vi "LoopselFF_1_or_2cam_eventdriven_CC3001.VI"() -> ()   [LabVIEW 2015]
uses:
  board.vis/Globals.vi
  <vilib>/Analysis/NI_AALBase.lvlib
panel:
  out "amount of devices":u8=1
  out "amount of cams":u8=1
  in  "CHB 8":bool
  in  "CHA 8":bool
  in  "CHB 7":bool
  in  "CHA 7":bool
  in  "CHB 6":bool
  in  "CHA 6":bool
  in  "CHB 5":bool
  in  "CHA 5":bool
  in  "CHB 4":bool
  in  "CHA 4":bool
  in  "CHB 3":bool
  in  "CHA 3":bool
  in  "CHB 2":bool
  in  "CHA 2":bool
  in  "CHB 1":bool
  in  "CHA 1":bool=TRUE
  in  "channel quick select (in hex)":u16=1 format="%x"
  out "tRMS":dbl=8.272957184592048 format="%0#.1f"
  out "mean":dbl=3064.5285285285286 format="%#_4f"
  in  "rms_pixel":u16=100
  in  "is FFT":bool=TRUE
  in  "IR gain":bool
  in  "continuous":bool=TRUE
  out "curr.block":u8=1
  out "Measure ON":bool
  in  "Board select\n1: board 1\n2: board 2\n3: both boards":u8=3
  in  "no.of blocks (nob)\npress enter":u32=1
  in  "block":u32(slide)=1 max=10 scale=0.9..1.0
  out "Signalverlaufgraph 2":u16[](graph)=[0, 0, 543, 543, 0, 1, 0, 0, 2, 2, 3, 3, 4, 4, 5, 5, 6, 6, 7, 7, 8, 8, 9, 9, 10, 10, 11, 11, 12, 12, 13, 13, 14, 14, 15, 15, 16, 16, 17, 17, 18, 18, 19, 19, 20, 20, 21, 21, 22, 22, 23, 23, 24, 24, 25, 25, 26, 26, 27, 27, 28, 28, 29, 29, 30, 30, 31, 31, 32, 32, 33, 33, 34, 34, 35, 35, 36, 36, 37, 37, 38, 38, 39, 39, 40, 40, 41, 41, 42, 42, 43, 43, 44, 44, 45, 45, 46, 46, 47, 47, 48, 48, 49, 49, 50, 50, 51, 51, 52, 52, 53, 53, 54, 54, 55, 55, 56, 56, 57, 57, 58, 58, 59, 59, 60, 60, 61, 61, 62, 62, 63, 63, 64, 64, 65, 65, 66, 66, 67, 67, 68, 68, 69, 69, 70, 70, 71, 71, 72, 72, 73, 73, 74, 74, 75, 75, 76, 76, 77, 77, 78, 78, 79, 79, 80, 80, 81, 81, 82, 82, 83, 83, 84, 84, 85, 85, 86, 86, 87, 87, 88, 88, 89, 89, 90, 90, 91, 91, 92, 92, 93, 93, 94, 94, 95, 95, 96, 96, 97, 97, 98, 98, 99, 99, 100, 100, 101, 101, 102, 102, 103, 103, 104, 104, 105, 105, 106, 106, 107, 107, 108, 108, 109, 109, 110, 110, 111, 111, 112, 112, 113, 113, 114, 114, 115, 115, 116, 116, 117, 117, 118, 118, 119, 119, 120, 120, 121, 121, 122, 122, 123, 123, 124, 124, 125, 125, 126, 126, 127, 127, 128, 128, 129, 129, 130, 130, 131, 131, 132, 132, 133, 133, 134, 134, 135, 135, 136, 136, 137, 137, 138, 138, 139, 139, 140, 140, 141, 141, 142, 142, 143, 143, 144, 144, 145, 145, 146, 146, 147, 147, 148, 148, 149, 149, 150, 150, 151, 151, 152, 152, 153, 153, 154, 154, 155, 155, 156, 156, 157, 157, 158, 158, 159, 159, 160, 160, 161, 161, 162, 162, 163, 163, 164, 164, 165, 165, 166, 166, 167, 167, 168, 168, 169, 169, 170, 170, 171, 171, 172, 172, 173, 173, 174, 174, 175, 175, 176, 176, 177, 177, 178, 178, 179, 179, 180, 180, 181, 181, 182, 182, 183, 183, 184, 184, 185, 185, 186, 186, 187, 187, 188, 188, 189, 189, 190, 190, 191, 191, 192, 192, 193, 193, 194, 194, 195, 195, 196, 196, 197, 197, 198, 198, 199, 199, 200, 200, 201, 201, 202, 202, 203, 203, 204, 204, 205, 205, 206, 206, 207, 207, 208, 208, 209, 209, 210, 210, 211, 211, 212, 212, 213, 213, 214, 214, 215, 215, 216, 216, 217, 217, 218, 218, 219, 219, 220, 220, 221, 221, 222, 222, 223, 223, 224, 224, 225, 225, 226, 226, 227, 227, 228, 228, 229, 229, 230, 230, 231, 231, 232, 232, 233, 233, 234, 234, 235, 235, 236, 236, 237, 237, 238, 238, 239, 239, 240, 240, 241, 241, 242, 242, 243, 243, 244, 244, 245, 245, 246, 246, 247, 247, 248, 248, 249, 249, 250, 250, 251, 251, 252, 252, 253, 253, 254, 254, 255, 255, 256, 256, 257, 257, 258, 258, 259, 259, 260, 260, 261, 261, 262, 262, 263, 263, 264, 264, 265, 265, 266, 266, 267, 267, 268, 268, 269, 269, 270, 270, 271, 271, 272, 272, 273, 273, 274, 274, 275, 275, 276, 276, 277, 277, 278, 278, 279, 279, 280, 280, 281, 281, 282, 282, 283, 283, 284, 284, 285, 285, 286, 286, 287, 287, 288, 288, 289, 289, 290, 290, 291, 291, 292, 292, 293, 293, 294, 294, 295, 295, 296, 296, 297, 297, 298, 298, 299, 299, 300, 300, 301, 301, 302, 302, 303, 303, 304, 304, 305, 305, 306, 306, 307, 307, 308, 308, 309, 309, 310, 310, 311, 311, 312, 312, 313, 313, 314, 314, 315, 315, 316, 316, 317, 317, 318, 318, 319, 319, 320, 320, 321, 321, 322, 322, 323, 323, 324, 324, 325, 325, 326, 326, 327, 327, 328, 328, 329, 329, 330, 330, 331, 331, 332, 332, 333, 333, 334, 334, 335, 335, 336, 336, 337, 337, 338, 338, 339, 339, 340, 340, 341, 341, 342, 342, 343, 343, 344, 344, 345, 345, 346, 346, 347, 347, 348, 348, 349, 349, 350, 350, 351, 351, 352, 352, 353, 353, 354, 354, 355, 355, 356, 356, 357, 357, 358, 358, 359, 359, 360, 360, 361, 361, 362, 362, 363, 363, 364, 364, 365, 365, 366, 366, 367, 367, 368, 368, 369, 369, 370, 370, 371, 371, 372, 372, 373, 373, 374, 374, 375, 375, 376, 376, 377, 377, 378, 378, 379, 379, 380, 380, 381, 381, 382, 382, 383, 383, 384, 384, 385, 385, 386, 386, 387, 387, 388, 388, 389, 389, 390, 390, 391, 391, 392, 392, 393, 393, 394, 394, 395, 395, 396, 396, 397, 397, 398, 398, 399, 399, 400, 400, 401, 401, 402, 402, 403, 403, 404, 404, 405, 405, 406, 406, 407, 407, 408, 408, 409, 409, 410, 410, 411, 411, 412, 412, 413, 413, 414, 414, 415, 415, 416, 416, 417, 417, 418, 418, 419, 419, 420, 420, 421, 421, 422, 422, 423, 423, 424, 424, 425, 425, 426, 426, 427, 427, 428, 428, 429, 429, 430, 430, 431, 431, 432, 432, 433, 433, 434, 434, 435, 435, 436, 436, 437, 437, 438, 438, 439, 439, 440, 440, 441, 441, 442, 442, 443, 443, 444, 444, 445, 445, 446, 446, 447, 447, 448, 448, 449, 449, 450, 450, 451, 451, 452, 452, 453, 453, 454, 454, 455, 455, 456, 456, 457, 457, 458, 458, 459, 459, 460, 460, 461, 461, 462, 462, 463, 463, 464, 464, 465, 465, 466, 466, 467, 467, 468, 468, 469, 469, 470, 470, 471, 471, 472, 472, 473, 473, 474, 474, 475, 475, 476, 476, 477, 477, 478, 478, 479, 479, 480, 480, 481, 481, 482, 482, 483, 483, 484, 484, 485, 485, 486, 486, 487, 487, 488, 488, 489, 489, 490, 490, 491, 491, 492, 492, 493, 493, 494, 494, 495, 495, 496, 496, 497, 497, 498, 498, 499, 499, 500, 500, 501, 501, 502, 502, 503, 503, 504, 504, 505, 505, 506, 506, 507, 507, 508, 508, 509, 509, 510, 510, 511, 511, 512, 512, 513, 513, 514, 514, 515, 515, 516, 516, 517, 517, 518, 518, 519, 519, 520, 520, 521, 521, 522, 522, 523, 523, 524, 524, 525, 525, 526, 526, 527, 527, 528, 528, 529, 529, 530, 530, 531, 531, 532, 532, 533, 533, 534, 534, 535, 535, 536, 536, 537, 537, 538, 538, 539, 539, 540, 540, 541, 541]
  out "Signalverlaufgraph":u16[](graph)=[2357, 2347, 2353, 2358, 0, 1, 0, 1, 2411, 2350, 2363, 2362, 2360, 34762, 35034, 35066, 35068, 35077, 35067, 35071, 35078, 35087, 35089, 35073, 35080, 35063, 35067, 35068, 35056, 35053, 35026, 35070, 35060, 35052, 35055, 35054, 35023, 35040, 35048, 35039, 35058, 35037, 35044, 35031, 35053, 35025, 35066, 35061, 35050, 35073, 35076, 35083, 35075, 35070, 35075, 35085, 35086, 35080, 35089, 35095, 35070, 35081, 35104, 35104, 35105, 35092, 35088, 35095, 35088, 35081, 35081, 35088, 35080, 35084, 35070, 35082, 35073, 35056, 35058, 35059, 35053, 35054, 35077, 35067, 35059, 35054, 35062, 35059, 35059, 35062, 35066, 35064, 35074, 35065, 35068, 35067, 35064, 35069, 35062, 35075, 35092, 35065, 35066, 35083, 35080, 35080, 35081, 35105, 35099, 35081, 35093, 35095, 35085, 35101, 35101, 35088, 35100, 35088, 35099, 35088, 35085, 35101, 35074, 35079, 35081, 35069, 35058, 35069, 35068, 35075, 35079, 35072, 35080, 35080, 35067, 35078, 35064, 35073, 35063, 35054, 35076, 35075, 35084, 35082, 35085, 35067, 35059, 35082, 35080, 35097, 35083, 35088, 35093, 35097, 35078, 35088, 35097, 35091, 35100, 35088, 35091, 35092, 35100, 35086, 35085, 35097, 35088, 35086, 35079, 35077, 35080, 35089, 35073, 35075, 35083, 35074, 35085, 35070, 35078, 35081, 35070, 35060, 35084, 35077, 35080, 35075, 35069, 35069, 35061, 35065, 35065, 35085, 35071, 35088, 35086, 35088, 35089, 35090, 35091, 35088, 35079, 35100, 35098, 35102, 35082, 35075, 35088, 35079, 35086, 35082, 35098, 35088, 35092, 35085, 35085, 35084, 35097, 35085, 35074, 35072, 35085, 35088, 35079, 35079, 35080, 35085, 35094, 35077, 35090, 35081, 35083, 35089, 35090, 35083, 35083, 35086, 35087, 35083, 35094, 35098, 35093, 35103, 35102, 35089, 35096, 35096, 35078, 35075, 35103, 35084, 35089, 35095, 35093, 35085, 35094, 35090, 35100, 35080, 35099, 35081, 35086, 35095, 35101, 35083, 35090, 35087, 35078, 35096, 35077, 35091, 35102, 35089, 35093, 35100, 35081, 35086, 35088, 35093, 35079, 35088, 35083, 35083, 35100, 35107, 35081, 35096, 35098, 35091, 35098, 35106, 35087, 35107, 35094, 35101, 35099, 35085, 35088, 35093, 35084, 35089, 35100, 35096, 35094, 35099, 35085, 35094, 35089, 35104, 35088, 35103, 35099, 35088, 35088, 35083, 35092, 35097, 35096, 35095, 35098, 35076, 35100, 35091, 35084, 35090, 35100, 35110, 35101, 35071, 35094, 35088, 35097, 35076, 35103, 35100, 35102, 35101, 35094, 35096, 35103, 35088, 35093, 35099, 35099, 35102, 35099, 35104, 35089, 35085, 35094, 35110, 35093, 35109, 35094, 35101, 35088, 35100, 35090, 35088, 35090, 35086, 35093, 35107, 35091, 35099, 35104, 35088, 35093, 35093, 35098, 35097, 35108, 35087, 35107, 35092, 35094, 35098, 35097, 35092, 35093, 35085, 35095, 35102, 35094, 35093, 35115, 35088, 35106, 35079, 35105, 35099, 35091, 35128, 35094, 35089, 35088, 35109, 35110, 35087, 35110, 35096, 35095, 35097, 35091, 35099, 35085, 35087, 35112, 35089, 35102, 35085, 35089, 35106, 35094, 35097, 35113, 35110, 35087, 35105, 35097, 35094, 35097, 35097, 35098, 35112, 35092, 35101, 35106, 35092, 35094, 35085, 35107, 35088, 35089, 35094, 35081, 35094, 35103, 35107, 35097, 35101, 35086, 35094, 35108, 35086, 35098, 35102, 35102, 35096, 35080, 35085, 35100, 35089, 35088, 35104, 35112, 35100, 35102, 35102, 35097, 35106, 35099, 35081, 35097, 35101, 35109, 35100, 35114, 35098, 35092, 32940, 29697, 29585, 29528, 29434, 29346, 29303, 29248, 29143, 29102, 29112, 29035, 28966, 28956, 28848, 28789, 28725, 28651, 28612, 28562, 28516, 28427, 28371, 28320, 28264, 28200, 28178, 28101, 28056, 27957, 27925, 27901, 27776, 27758, 27701, 27631, 27579, 27545, 27475, 27425, 27382, 27318, 27302, 27222, 27176, 27114, 27069, 27020, 26974, 26944, 26887, 26793, 26807, 26744, 26714, 26624, 26586, 26540, 26466, 26393, 26379, 26282, 26220, 26157, 26029, 25929, 25768, 25543, 2252, 2400, 2386, 2390, 2368, 2373, 2377, 2379, 2379, 2378, 2377, 2380, 2373, 2379, 2386, 2383, 2376, 2381, 2378, 2377, 2376, 2373, 2385, 2377, 2381, 2376, 2379, 2379, 2376, 2376, 2376, 2379, 2384, 2378, 2374, 2380, 2377, 2381, 2380, 2371, 2379, 2376, 2379, 2384, 2380, 2380, 2377, 2368, 2376, 2375, 2378, 2370, 2374, 2375, 2383, 2372, 2379, 2374, 2381, 2369, 2375, 2368, 2373, 2368, 2368, 2372, 2374, 2371, 2368, 2373, 2372, 2370, 2372, 2374, 2375, 2367, 2367, 2370, 2369, 2375, 2372, 2373, 2378, 2372, 2366, 2372, 2370, 2374, 2365, 2373, 2375, 2374, 2370, 2370, 2369, 2369, 2374, 2371, 2373, 2371, 2372, 2371, 2366, 2368, 2370, 2362, 2370, 2372, 2366, 2374, 2369, 2368, 2371, 2368, 2365, 2362, 2375, 2373, 2369, 2366, 2367, 2371, 2362, 2377, 2371, 2367, 2369, 2366, 2371, 2366, 2364, 2366, 2360, 2365, 2374, 2362, 2371, 2373, 2366, 2364, 2367, 2364, 2368, 2360, 2360, 2363, 2367, 2368, 2367, 2371, 2364, 2368, 2366, 2359, 2363, 2365, 2368, 2368, 2358, 2357, 2365, 2364, 2369, 2362, 2364, 2364, 2363, 2358, 2363, 2364, 2359, 2360, 2358, 2370, 2358, 2361, 2363, 2355, 2361, 2369, 2363, 2366, 2365, 2368, 2363, 2360, 2359, 2361, 2359, 2363, 2356, 2365, 2362, 2360, 2368, 2362, 2366, 2370, 2358, 2366, 2364, 2366, 2362, 2363, 2356, 2365, 2363, 2361, 2363, 2367, 2366, 2365, 2357, 2366, 2359, 2361, 2360, 2360, 2363, 2365, 2364, 2360, 2360, 2357, 2355, 2362, 2361, 2361, 2364, 2364, 2361, 2364, 2361, 2363, 2358, 2363, 2357, 2355, 2357, 2365, 2357, 2367, 2365, 2363, 2354, 2360, 2356, 2358, 2362, 2359, 2360, 2362, 2362, 2355, 2360, 2360, 2360, 2361, 2360, 2359, 2357, 2364, 2359, 2361, 2362, 2360, 2359, 2360, 2355, 2355, 2362, 2358, 2358, 2357, 2357, 2360, 2360, 2363, 2353, 2353, 2358, 2358, 2358, 2362, 2360, 2362, 2359, 2356, 2357, 2360, 2355, 2353, 2360, 2362, 2358, 2358, 2350, 2357, 2362, 2354, 2354, 2356, 2360, 2360, 2355, 2361, 2354, 2360, 2356, 2355, 2355, 2362, 2359, 2362, 2363, 2359, 2361, 2358, 2355, 2356, 2354, 2358, 2364, 2356, 2362, 2358, 2354, 2360, 2362, 2361, 2358, 2361, 2362, 2358, 2363, 2359, 2363, 2364, 2356, 2357, 2356, 2354, 2360, 2357, 2355, 2359, 2358, 2356, 2362, 2360, 2357, 2359, 2357, 2357, 2355, 2357, 2357, 2357, 2364, 2360, 2355, 2358, 2355, 2357, 2360, 2353, 2355, 2352, 2362, 2354, 2355, 2360, 2357, 2352, 2359, 2356, 2356, 2358, 2353, 2357, 2356, 2355, 2349, 2361, 2358, 2354, 2358, 2359, 2355, 2360, 2354, 2357, 2357, 2353, 2354, 2359, 2359, 2355, 2349, 2358, 2358, 2355, 2353, 2353, 2357, 2357, 2357, 2354, 2358, 2359, 2354, 2353, 2352, 2358, 2361, 2357, 2350, 2350, 2352, 2360, 2351, 2355, 2354, 2360, 2357, 2355, 2355, 2355, 2350, 2357, 2357, 2358, 2358, 2356, 2353, 2352, 2354, 2353, 2357, 2357, 2353, 2358, 2360, 2361, 2355, 2357, 2361, 2357, 2358, 2356, 2355, 2358, 2354, 2351, 2355, 2352, 2354, 2352, 2354, 2363, 2359, 2358, 2357, 2349, 2358, 2352, 2356, 2355, 2359, 2353, 2353, 2361, 2359, 2359, 2357, 2357, 2349, 2353, 2353, 2350, 2358, 2357, 2356, 2358, 2356, 2356, 2355, 2355, 2355, 2351, 2355, 2357, 2352, 2354, 2348, 2354, 2348, 2354, 2350, 2352, 2353, 2359, 2356, 2351, 2356, 2357, 2352, 2354, 2355, 2359, 2353, 2354, 2352, 2349, 2362, 2353, 2360, 2349, 2357, 2352, 2359, 2348, 2359, 2349, 2358, 2348, 2349, 2351, 2356, 2353, 2358, 2353, 2354, 2360, 2355, 2356, 2358, 2348, 2351, 2354, 2358, 2360, 2360, 2359, 2356, 2356, 2354, 2357, 2350, 2351, 2351]
  out "boards recognised":u8=1
  in  "alloc mem":bool
  out "FREE \nRAM MB":dbl=14941.0
  out "BUILT-IN\nRAM MB":dbl=18096.0
  out "SEC":dbl=5.9999999999999995e-05
  out "MB RAM":dbl
  in  "pos slope":u8=1
  in  "both slopes":u8
  in  "DAT in 10ns":u32
  in  "extTrig  0/1\n0 : internal\n1:  \"I\" input (laser)":u8
  in  "stop all":bool
  in  "start":bool
  in  "sample":u32(slide)=2 max=3000 scale=0.9..110.0
  in  "no.of samples (nos)":u32=3000
  in  "exposuretime[ms]":dbl=1.0 format="%.3f"
  # "Camera Control 1"
  # "Camera Control 5"
  # "Start with run"
  # "Abort with ESC"
  # "Camera Control 6"
  # "Camera Control 2"
  # "Camera Control 3"
  # "Camera Control 7"
  # "Camera Control 4"
  # "Camera Control 8"
  # "press Esc to stop measurement"
  # "exit here"
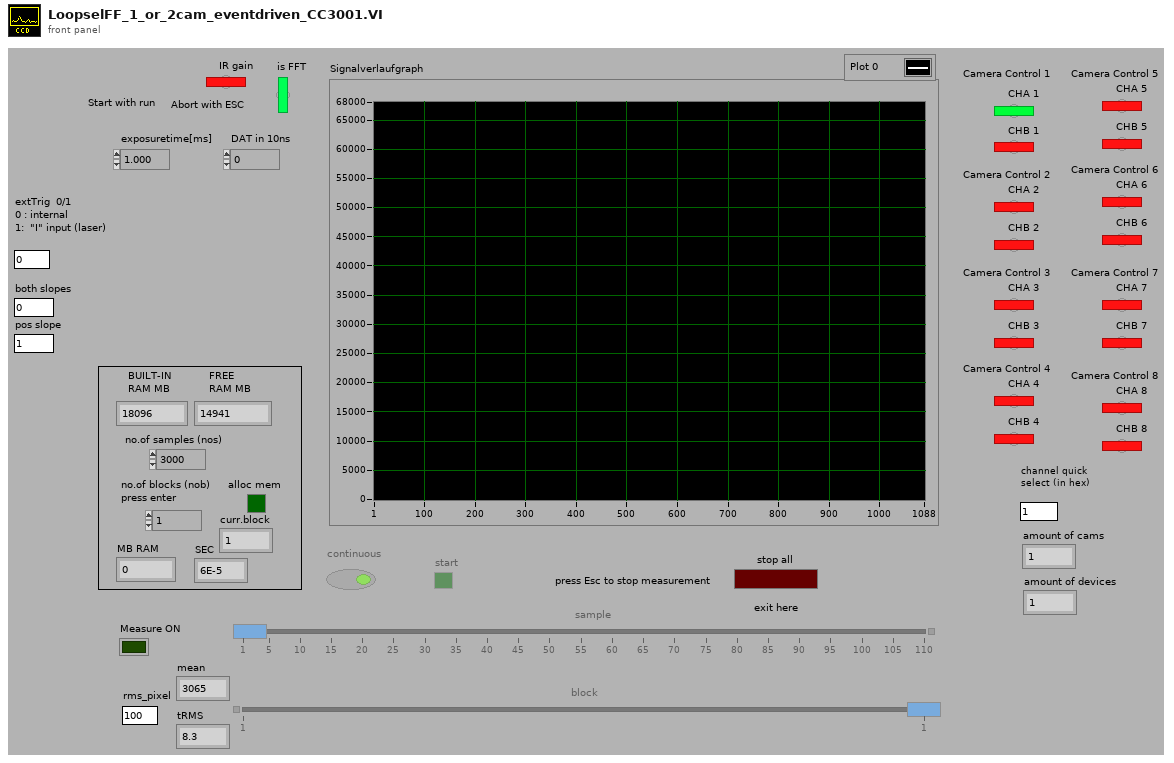
[diagram p1: front panel]
types:
  T1 = enum8{"Enabled", "Disabled", "Disabled and Grayed Out"}
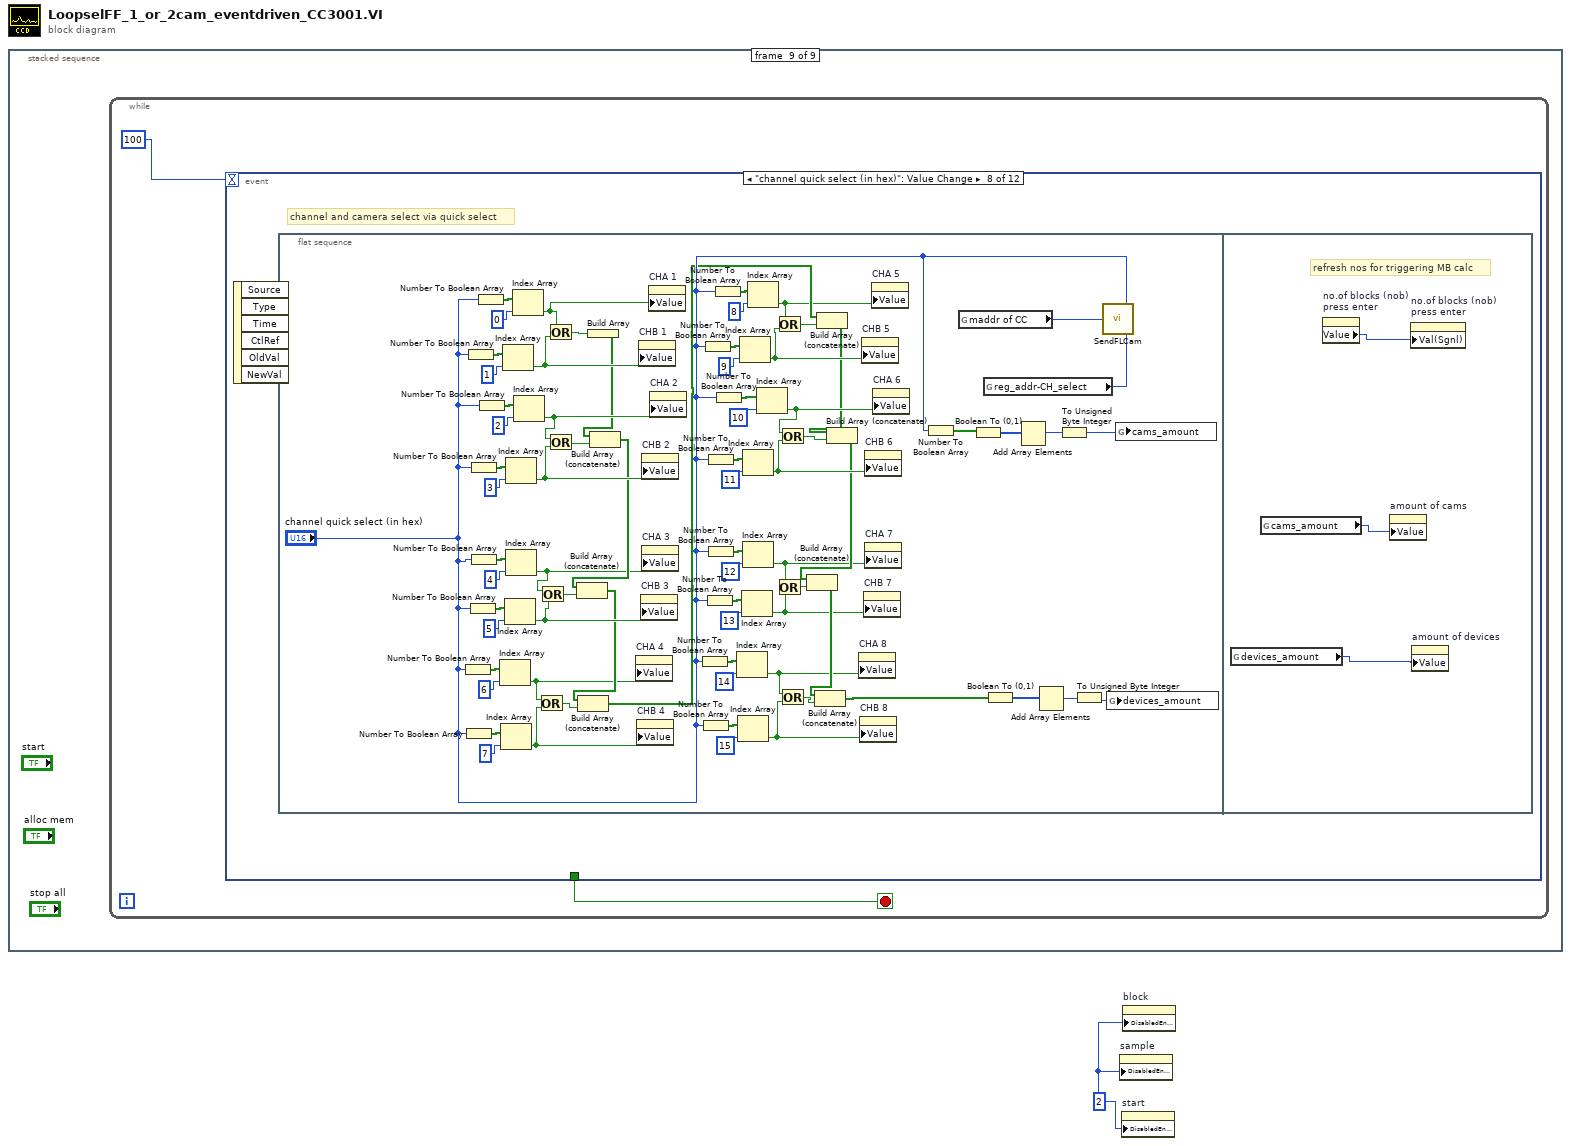
[diagram p0: block diagram]
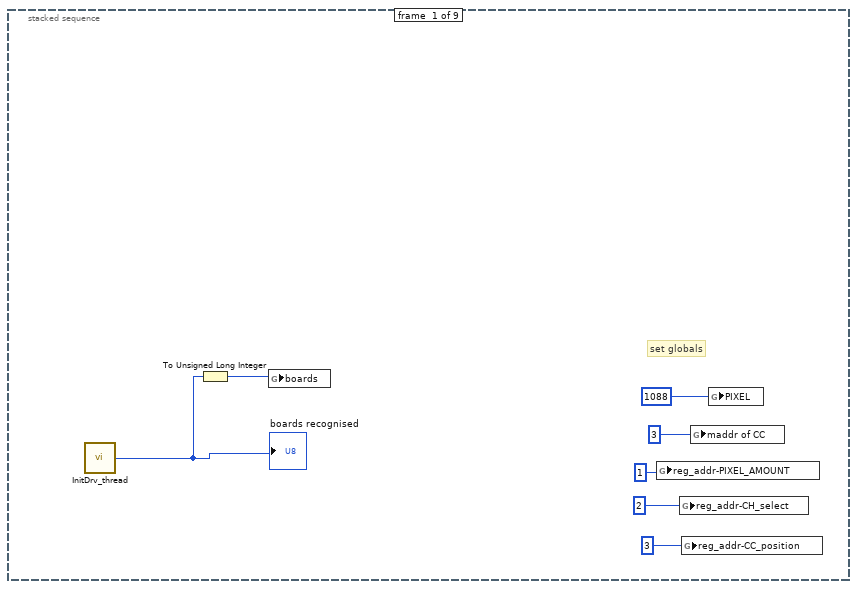
[diagram p2: hidden frame]
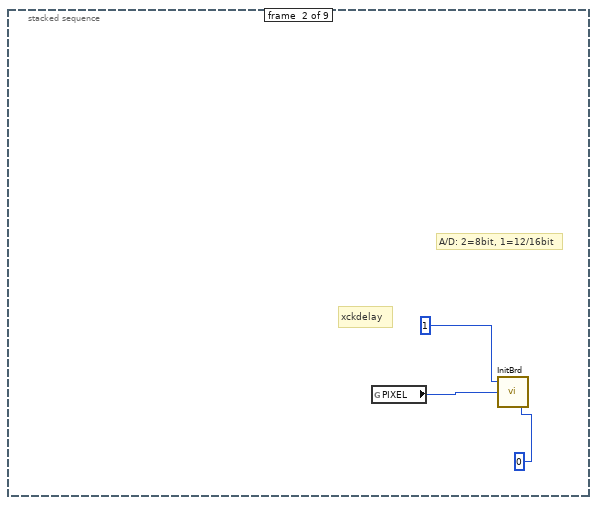
[diagram p3: hidden frame]
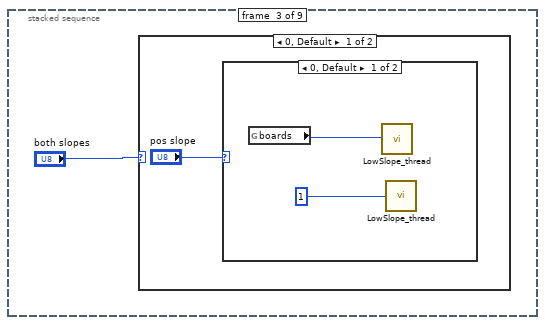
[diagram p4: hidden frame]
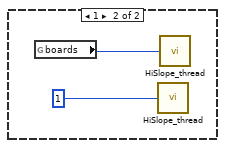
[diagram p5: hidden frame]
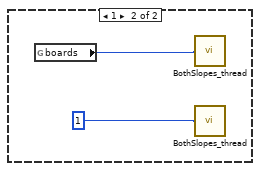
[diagram p6: hidden frame]
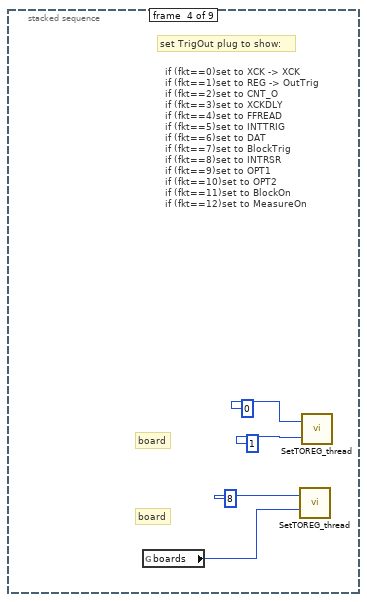
[diagram p7: hidden frame]
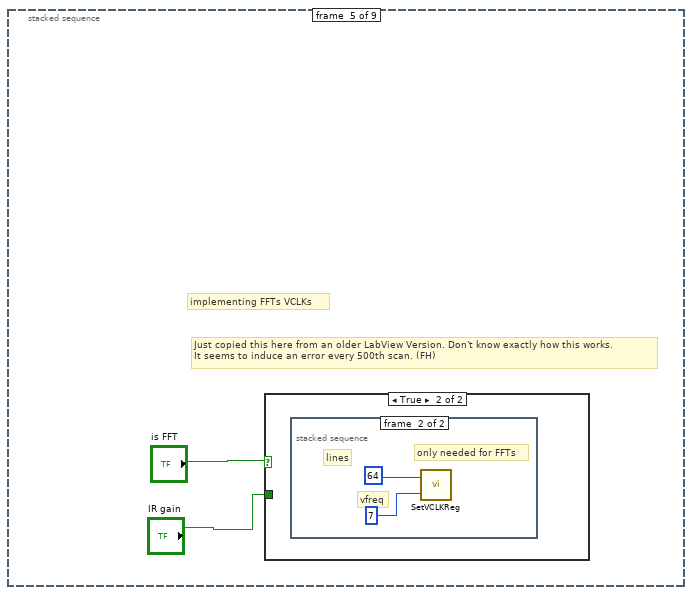
[diagram p8: hidden frame]
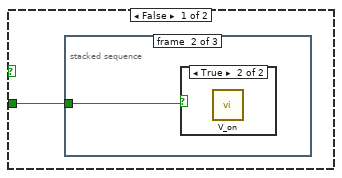
[diagram p9: hidden frame]
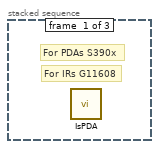
[diagram p10: hidden frame]
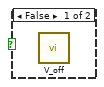
[diagram p11: hidden frame]
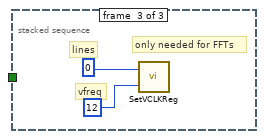
[diagram p12: hidden frame]
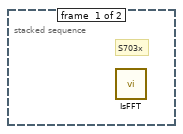
[diagram p13: hidden frame]
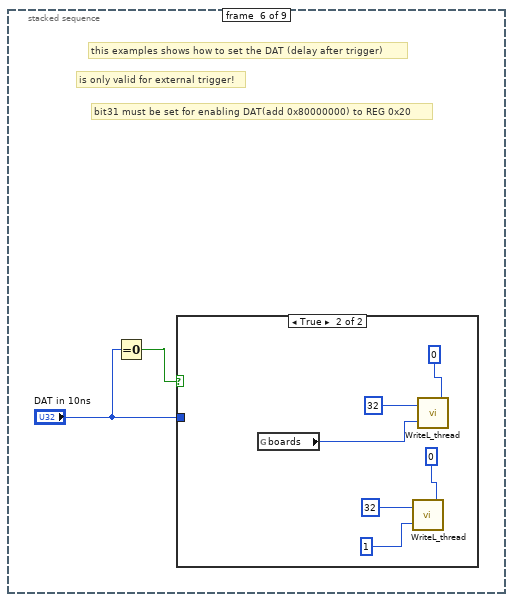
[diagram p14: hidden frame]
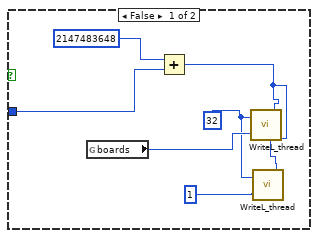
[diagram p15: hidden frame]
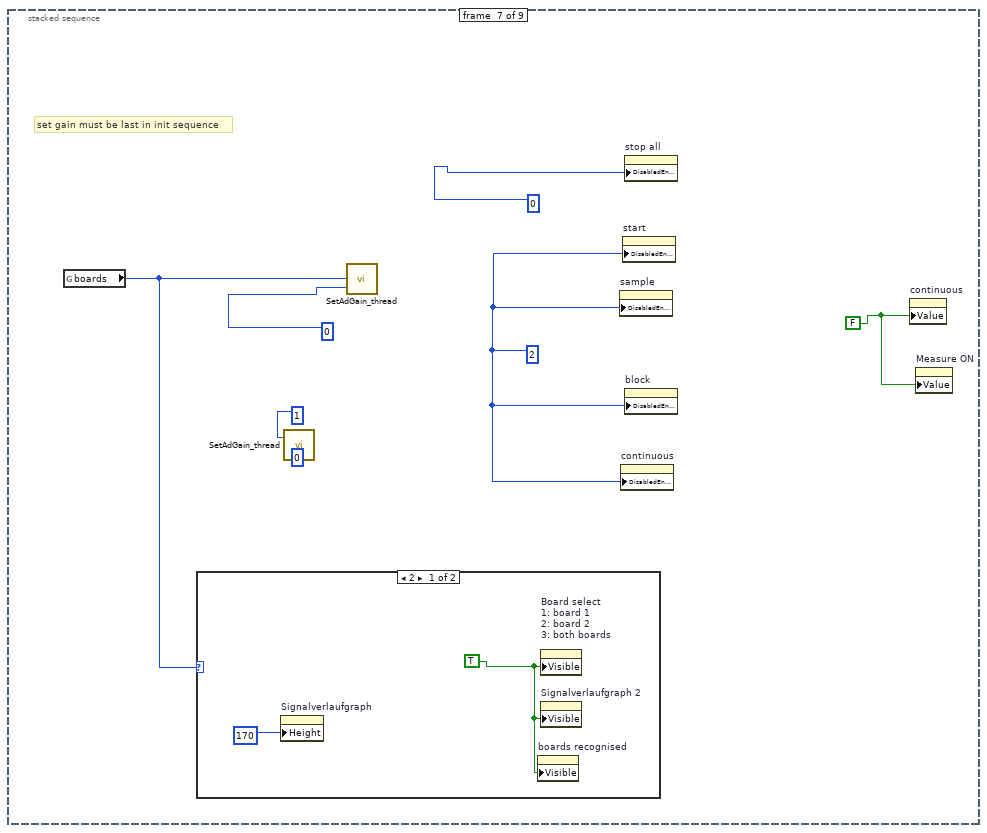
[diagram p16: hidden frame]
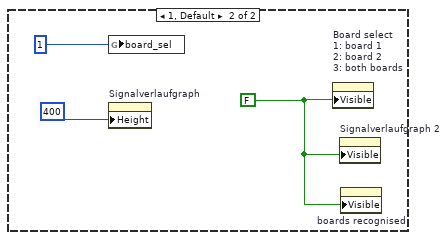
[diagram p17: hidden frame]
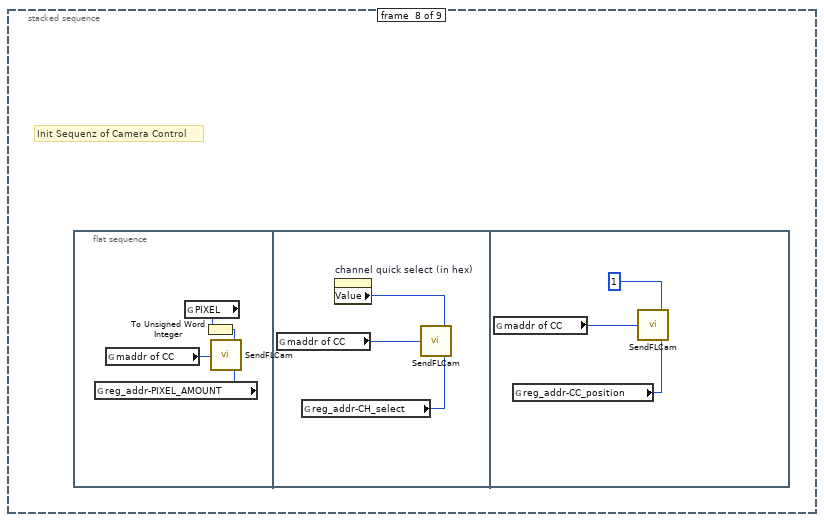
[diagram p18: hidden frame]
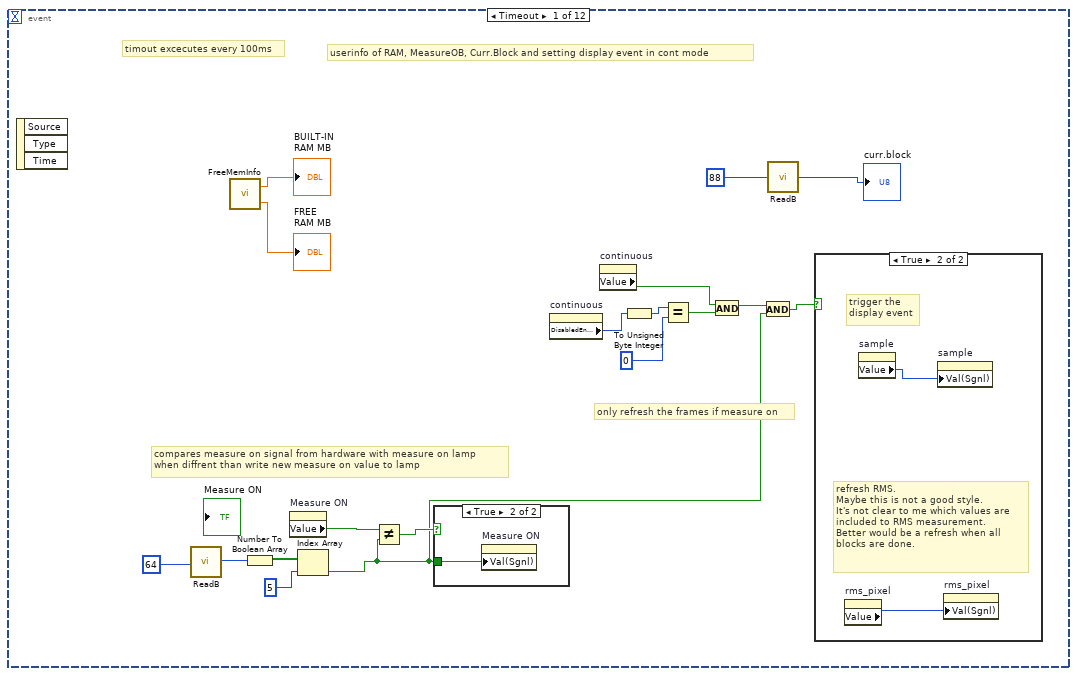
[diagram p19: hidden frame]
diagram:
  w1 = 2
  n1 = stacked-sequence {
    frame #0 {
      # "set globals"
      n2 = call "InitDrv_thread.vi"() -> ("Boards"=w6:u8)  [unwired: 1 in]
      "boards recognised" <- w6
      n3 = To Unsigned Long Integer(number=w6) -> (unsigned 32bit integer=w7:u32)
      n4 = global write "Globals.vi" "boards"(w7) -> ()
      n5 = global write "Globals.vi" "reg_addr-PIXEL_AMOUNT"(u8 1) -> ()
      n6 = global write "Globals.vi" "reg_addr-CH_select"(u8 2) -> ()
      n7 = global write "Globals.vi" "reg_addr-CC_position"(u8 3) -> ()
      n8 = global write "Globals.vi" "maddr of CC"(u8 3) -> ()
      n9 = global write "Globals.vi" "PIXEL"(u32 1088) -> ()
    }
    frame #1 {
      # "xckdelay"
      # "A/D: 2=8bit, 1=12/16bit"
      n10 = global read "Globals.vi" "PIXEL"() -> (w11:u32)
      n11 = call "InitBrd.vi"("xckdly"=u32 0, "pixel"=w11, "flag816"=u32 1) -> ()  [unwired: 3 in]
    }
    frame #2 {
      n12 = case shown="0, Default" "both slopes" {
        frame 0, Default {
          n13 = case shown="0, Default" "pos slope" {
            frame 0, Default {
              n14 = global read "Globals.vi" "boards"() -> (w14:u32)
              n15 = call "LowSlope_thread.vi"("board"=w14) -> ()  [unwired: 1 in]
              n16 = call "LowSlope_thread.vi"("board"=1) -> ()  [unwired: 1 in]
            }
            frame 1 {
              n17 = global read "Globals.vi" "boards"() -> (w17:u32)
              n18 = call "HiSlope_thread.vi"("board"=1) -> ()  [unwired: 1 in]
              n19 = call "HiSlope_thread.vi"("board"=w17) -> ()  [unwired: 1 in]
            }
          }
        }
        frame 1 {
          n20 = global read "Globals.vi" "boards"() -> (w19:u32)
          n21 = call "BothSlopes_thread.vi"("board"=w19) -> ()  [unwired: 1 in]
          n22 = call "BothSlopes_thread.vi"("board"=1) -> ()  [unwired: 1 in]
        }
      }
    }
    frame #3 {
      # "board"
      # "board"
      # "set TrigOut plug to show:"
      # "if (fkt==0)set to XCK -> XCK\nif (fkt==1)set to REG -> OutTrig\nif (fkt==2)set to CNT_O\nif (fkt==3)set to XCKDLY\nif (fkt==4)set to FFREAD\nif (fkt==5)set to INTTRIG\nif (fkt==6)set to DAT\nif (fkt==7)set to BlockTrig\nif (fkt==8)set to INTRSR\nif (fkt==9)set to OPT1\nif (fkt==10)set to OPT2\nif (fkt==11)set to BlockOn\nif (fkt==12)set to MeasureOn"
      n23 = global read "Globals.vi" "boards"() -> (w23:u32)
      n24 = call "SetTOREG_thread.vi"("board"=w23, "fkt"=u8 8) -> ()  [unwired: 1 in]
      n25 = call "SetTOREG_thread.vi"("board"=u32 1, "fkt"=u8 0) -> ()  [unwired: 1 in]
    }
    frame #4 {
      # "implementing FFTs VCLKs"
      # "Just copied this here from an older LabView Version. Don't know exactly how this works.\nIt seems to induce an error every 500th scan. (FH)"
      n26 = case shown="True" "is FFT" {
        tunnel: "IR gain" -> [w26 _]
        frame False {
          n27 = stacked-sequence {
            tunnel: w26 -> [_ w27 _]
            frame #0 {
              # "For IRs G11608"
              # "For PDAs S390x"
              n28 = call "IsPDA.vi"() -> ()  [unwired: 1 in]
            }
            frame #1 {
              n29 = case shown="True" w27 {
                frame False {
                  n30 = call "V_off.vi"() -> ()  [unwired: 1 in]
                }
                frame True {
                  n31 = call "V_on.vi"() -> ()  [unwired: 1 in]
                }
              }
            }
            frame #2 {
              # "only needed for FFTs"
              # "vfreq"
              # "lines"
              n32 = call "SetVCLKReg.vi"("vfreq"=u8 12, "lines"=u32 0) -> ()  [unwired: 1 in]
            }
          }
        }
        frame True {
          n33 = stacked-sequence {
            frame #0 {
              # "S703x"
              n34 = call "IsFFT.vi"() -> ()  [unwired: 1 in]
            }
            frame #1 {
              # "only needed for FFTs"
              # "vfreq"
              # "lines"
              n35 = call "SetVCLKReg.vi"("vfreq"=u8 7, "lines"=u32 64) -> ()  [unwired: 1 in]
            }
          }
        }
      }
    }
    frame #5 {
      # "bit31 must be set for enabling DAT(add 0x80000000) to REG 0x20"
      # "is only valid for external trigger!"
      # "this examples shows how to set the DAT (delay after trigger)"
      n36 = Equal To 0?(x="DAT in 10ns") -> (x = 0?=w33:bool)
      n37 = case shown="True" w33 {
        tunnel: "DAT in 10ns" -> [w38 _]
        frame False {
          w35 = u32 32
          n38 = global read "Globals.vi" "boards"() -> (w37:u32)
          n39 = Add(x=u32 2147483648, y=w38) -> (x+y=w36:u32)
          n40 = call "WriteL_thread.vi"("val"=w36, "board"=w37, "offset"=w35) -> ()
          n41 = call "WriteL_thread.vi"("val"=w36, "board"=u32 1, "offset"=w35) -> ()
        }
        frame True {
          n42 = global read "Globals.vi" "boards"() -> (w44:u32)
          n43 = call "WriteL_thread.vi"("val"=u32 0, "board"=u32 1, "offset"=u32 32) -> ()
          n44 = call "WriteL_thread.vi"("val"=u32 0, "board"=w44, "offset"=u32 32) -> ()
        }
      }
    }
    frame #6 {
      w46 = FALSE
      w52 = 2
      # "set gain must be last in init sequence"
      n45 = global read "Globals.vi" "boards"() -> (w50:u32)
      n46 = case shown="2" w50 {
        frame 2 {
          w54 = TRUE
          n47 = property on="Signalverlaufgraph" class="WFGraph (strict)"("Height"=u8 170) -> ()  [unwired: 2 in, 2 out]
          n48 = property on="boards recognised" class="DigNum (strict)"("Visible"=w54) -> ()  [unwired: 2 in, 2 out]
          n49 = property on="Board select\n1: board 1\n2: board 2\n3: both boards" class="DigNum (strict)"("Visible"=w54) -> ()  [unwired: 2 in, 2 out]
          n50 = property on="Signalverlaufgraph 2" class="WFGraph (strict)"("Visible"=w54) -> ()  [unwired: 2 in, 2 out]
        }
        frame 1, Default {
          w55 = FALSE
          n51 = global write "Globals.vi" "board_sel"(u8 1) -> ()
          n52 = property on="Signalverlaufgraph" class="WFGraph (strict)"("Height"=400) -> ()  [unwired: 2 in, 2 out]
          n53 = property on="Board select\n1: board 1\n2: board 2\n3: both boards" class="DigNum (strict)"("Visible"=w55) -> ()  [unwired: 2 in, 2 out]
          n54 = property on="Signalverlaufgraph 2" class="WFGraph (strict)"("Visible"=w55) -> ()  [unwired: 2 in, 2 out]
          n55 = property on="boards recognised" class="DigNum (strict)"("Visible"=w55) -> ()  [unwired: 2 in, 2 out]
        }
      }
      n56 = call "SetAdGain_thread.vi"("gain"=u8 0, "board"=u32 1) -> ()  [unwired: 1 in]
      n57 = call "SetAdGain_thread.vi"("gain"=u8 0, "board"=w50) -> ()  [unwired: 1 in]
      n58 = property on="sample" class="Slide (strict)"("DisabledEnum"=w52) -> ()  [unwired: 2 in, 2 out]
      n59 = property on="continuous" class="Bool (strict)"("DisabledEnum"=w52) -> ()  [unwired: 2 in, 2 out]
      n60 = property on="start" class="Bool (strict)"("DisabledEnum"=w52) -> ()  [unwired: 2 in, 2 out]
      n61 = property on="stop all" class="Bool (strict)"("DisabledEnum"=0) -> ()  [unwired: 2 in, 2 out]
      n62 = property on="block" class="Slide (strict)"("DisabledEnum"=w52) -> ()  [unwired: 2 in, 2 out]
      n63 = property on="continuous" class="Bool (strict)"("Value"=w46) -> ()  [unwired: 2 in, 2 out]
      n64 = property on="Measure ON" class="Bool (strict)"("Value"=w46) -> ()  [unwired: 2 in, 2 out]
    }
    frame #7 {
      # "Init Sequenz of Camera Control"
      n65 = flat-sequence {
        frame #0 {
          n66 = global read "Globals.vi" "reg_addr-PIXEL_AMOUNT"() -> (w61:u8)
          n67 = global read "Globals.vi" "maddr of CC"() -> (w60:u8)
          n68 = global read "Globals.vi" "PIXEL"() -> (w59:u32)
          n69 = To Unsigned Word Integer(number=w59) -> (unsigned 16bit integer=w58:u16)
          n70 = call "SendFLCam.vi"("madr"=w60, "data"=w58, "adadr"=w61) -> ()
        }
        frame #1 {
          n71 = global read "Globals.vi" "maddr of CC"() -> (w64:u8)
          n72 = global read "Globals.vi" "reg_addr-CH_select"() -> (w63:u8)
          n73 = property on="channel quick select (in hex)" class="DigNum (strict)"() -> ("Value"=w62:u16)  [unwired: 2 in, 2 out]
          n74 = call "SendFLCam.vi"("madr"=w64, "data"=w62, "adadr"=w63) -> ()
        }
        frame #2 {
          n75 = global read "Globals.vi" "maddr of CC"() -> (w67:u8)
          n76 = global read "Globals.vi" "reg_addr-CC_position"() -> (w66:u8)
          n77 = call "SendFLCam.vi"("madr"=w67, "data"=u16 1, "adadr"=w66) -> ()
        }
      }
    }
    frame #8 {
      n78 = while {
        stop <- w69 stop-if-true
        n79 = event shown="[7] \"channel quick select (in hex)\": Value Change" {
          selector: _ -> [_ _ _ _ _ _ _ _ _ _ _ _]
          dyn-events: _ -> [_ _ _ _ _ _ _ _ _ _ _ _]
          timeout: 100 -> [_ _ _ _ _ _ _ _ _ _ _ _]
          tunnel: [_ _ _ _ _ _ _ _ _ _ w318 _] -> w69
          event Timeout {
            # "only refresh the frames if measure on"
            # "compares measure on signal from hardware with measure on lamp\nwhen diffrent than write new measure on value to lamp"
            # "timout excecutes every 100ms"
            # "userinfo of RAM, MeasureOB, Curr.Block and setting display event in cont mode"
            n80 = event-data() -> ()  [unwired: 1 in, 3 out]
            n81 = call "ReadB.vi"("Offset"=u32 64) -> ("Data"=w84:u8)
            n82 = call "FreeMemInfo.vi"() -> ("PhysicalSpace"=→"BUILT-IN\nRAM MB":dbl, "PhysicalFreeSpace"=→"FREE \nRAM MB":dbl)  [unwired: 1 in]
            n83 = Number To Boolean Array(number=w84) -> (Boolean array=w83:bool[])
            n84 = property on="Measure ON" class="Bool (strict)"() -> ("Value"=w77:bool)  [unwired: 2 in, 2 out]
            n85 = Index Array(array=w83, index=5) -> (element=w73:bool)
            n86 = Not Equal?(x=w77, y=w73) -> (x != y?=w76:bool)
            n87 = case shown="True" w76 {
              tunnel: w73 -> [_ w88]
              frame False {
              }
              frame True {
                n88 = property on="Measure ON" class="Bool (strict)"("Val(Sgnl)"=w88) -> ()  [unwired: 2 in, 2 out]
              }
            }
            n89 = property on="continuous" class="Bool (strict)"() -> ("DisabledEnum"=w70:T1)  [unwired: 2 in, 2 out]
            n90 = property on="continuous" class="Bool (strict)"() -> ("Value"=w79:bool)  [unwired: 2 in, 2 out]
            n91 = To Unsigned Byte Integer(number=w70) -> (unsigned 8bit integer=w71:u8)
            n92 = Equal?(x=w71, y=u8 0) -> (x = y?=w78:bool)
            n93 = And(x=w79, y=w78) -> (x .and. y?=w75:bool)
            n94 = And(x=w75, y=w73) -> (x .and. y?=w74:bool)
            n95 = call "ReadB.vi"("Offset"=u32 88) -> ("Data"=→"curr.block":u8)
            n96 = case shown="True" w74 {
              frame False {
              }
              frame True {
                # "refresh RMS.\nMaybe this is not a good style.\nIt's not clear to me which values are \nincluded to RMS measurement.\nBetter would be a refresh when all\nblocks are done."
                # "trigger the \ndisplay event"
                n97 = property on="rms_pixel" class="DigNum (strict)"() -> ("Value"=w89:u16)  [unwired: 2 in, 2 out]
                n98 = property on="sample" class="Slide (strict)"() -> ("Value"=w90:u32)  [unwired: 2 in, 2 out]
                n99 = property on="sample" class="Slide (strict)"("Val(Sgnl)"=w90) -> ()  [unwired: 2 in, 2 out]
                n100 = property on="rms_pixel" class="DigNum (strict)"("Val(Sgnl)"=w89) -> ()  [unwired: 2 in, 2 out]
              }
            }
          }
          event "Measure ON": Value Change {
            # "triggers on value change of measure on. this happens on start of measurement and after measurement\nwhen continuous: not after finishing all blocks, only when exiting measurement"
            n101 = event-data() -> ("NewVal"=w91:bool)  [unwired: 1 in, 5 out]
            n102 = property on="continuous" class="Bool (strict)"() -> ("Value"=w92:bool)  [unwired: 2 in, 2 out]
            n103 = And(x=w92, y=w91) -> (x .and. y?=w93:bool)
            n104 = case shown="False" w91 {
              frame False {
                n105 = property on="stop all" class="Bool (strict)"("DisabledEnum"=0) -> ()  [unwired: 2 in, 2 out]
              }
              frame True {
              }
            }
            n106 = case shown="True" w93 {
              frame False {
              }
              frame True {
                n107 = property on="stop all" class="Bool (strict)"("DisabledEnum"=2) -> ()  [unwired: 2 in, 2 out]
              }
            }
          }
          event "Board select\n1: board 1\n2: board 2\n3: both boards": Value Change {
            # "selecting number of cams"
            n108 = event-data() -> ()  [unwired: 1 in, 6 out]
            n109 = global read "Globals.vi" "boards"() -> (w96:u32)
            n110 = case shown="2" w96 {
              frame 0, Default {
              }
              frame 2 {
                n111 = global write "Globals.vi" "board_sel"("Board select\n1: board 1\n2: board 2\n3: both boards") -> ()
              }
            }
          }
          event "continuous": Value Change {
            # "setting continuos mode"
            n112 = event-data() -> ()  [unwired: 1 in, 6 out]
            n113 = case shown="False" "continuous" {
              tunnel: [u8 0 u8 1] -> w98
              frame False {
              }
              frame True {
              }
            }
            n114 = call "contFFLoop.vi"("Numeric"=w98) -> ()  [unwired: 1 in]
          }
          event "alloc mem": Value Change {
            w108 = 0
            # "update params"
            # "Setup DMA"
            n115 = event-data() -> ()  [unwired: 1 in, 6 out]
            n116 = global read "Globals.vi" "cams_amount"() -> (w105:u8)
            n117 = global read "Globals.vi" "nob"() -> (w106:u32)
            n118 = global read "Globals.vi" "nos"() -> (w107:u32)
            n119 = To Unsigned Long Integer(number=w105) -> (unsigned 32bit integer=w104:u32)
            n120 = global read "Globals.vi" "boards"() -> (w111:u32)
            n121 = Multiply(x=w104, y=w106) -> (x*y=w102:u32)
            n122 = Multiply(x=w104, y=w107) -> (x*y=w103:u32)
            n123 = case shown="2" w111 {
              selector: w111 -> [_ w112]
              tunnel: w103 -> [_ w113]
              tunnel: w102 -> [_ w114]
              frame 1, Default {
              }
              frame 2 {
                # "Setup DMA"
                n124 = call "SetupDMA_thread.vi"("blocks"=w114, "nos"=w113, "Drv"=w112) -> ()  [unwired: 2 in]
              }
            }
            n125 = call "SetupDMA_thread.vi"("blocks"=w102, "nos"=w103, "Drv"=u32 1) -> ()  [unwired: 2 in]
            n126 = property on="continuous" class="Bool (strict)"("DisabledEnum"=w108) -> ()  [unwired: 2 in, 2 out]
            n127 = property on="block" class="Slide (strict)"("DisabledEnum"=w108) -> ()  [unwired: 2 in, 2 out]
            n128 = property on="sample" class="Slide (strict)"("DisabledEnum"=w108) -> ()  [unwired: 2 in, 2 out]
            n129 = property on="exposuretime[ms]" class="DigNum (strict)"() -> ("Value"=w110:dbl)  [unwired: 2 in, 2 out]
            n130 = property on="start" class="Bool (strict)"("DisabledEnum"=w108) -> ()  [unwired: 2 in, 2 out]
            n131 = property on="exposuretime[ms]" class="DigNum (strict)"("Val(Sgnl)"=w110) -> ()  [unwired: 2 in, 2 out]
          }
          event "start": Mouse Down {
            # "start measurement"
            # "only 1st PCI board is used for ext. trig."
            # "ext. block trig\n0: internal: Space\n1: PCI \"I\"\n2: S1\n3: S2"
            # "block trigger 0/1\n0: internal -> next block is started immediately \n1: external -> each block has an own trigger"
            n132 = event-data() -> ()  [unwired: 1 in, 8 out]
            n133 = global read "Globals.vi" "exp time"() -> (w120:dbl)
            n134 = Multiply(x=1000.0, y=w120) -> (x*y=w122:dbl)
            n135 = global read "Globals.vi" "board_sel"() -> (w115:u8)
            n136 = To Unsigned Long Integer(number=w122) -> (unsigned 32bit integer=w117:u32)
            n137 = call "ReadFFLoop_thread.vi"("blocktrigger"=u8 0, "btrig_ch"=u8 0, "ExtTrig"="extTrig  0/1\n0 : internal\n1:  \"I\" input (laser)", "cam_sel"=w115, "exptus"=w117) -> ()  [unwired: 1 in]
          }
          event "sample", "block": Value Change {
            w134 = u32 1
            # "when selecting a value\nbigger than possible\nnos or nob, a dummy \nvalue \"1\" is chosen\n\nTODO:\ninsert error handling\nwith lower values than 1"
            # "display"
            n138 = event-data() -> ()  [unwired: 1 in, 6 out]
            n139 = global read "Globals.vi" "boards"() -> (w137:u32)
            n140 = global read "Globals.vi" "nob"() -> (w126:u32)
            n141 = global read "Globals.vi" "nos"() -> (w133:u32)
            n142 = Greater?(x=w126, y="block") -> (0:w129:bool)
            n143 = Greater?(x=w133, y="sample") -> (0:w132:bool)
            n144 = global read "Globals.vi" "PIXEL"() -> (w123:u32)
            n145 = case shown="False" w129 {
              tunnel: [u32 1 w142] -> w128
              tunnel: "block" -> [_ w142]
              frame False {
              }
              frame True {
              }
            }
            n146 = case shown="False" w132 {
              tunnel: [u32 1 w144] -> w131
              tunnel: "sample" -> [_ w144]
              frame False {
              }
              frame True {
              }
            }
            n147 = To Long Integer(number=w123) -> (32bit integer=w124:i32)
            n148 = Initialize Array(u16 100, w124) -> (w140:u16[])
            n149 = Subtract(x=w131, y=w134) -> (x-y=w136:u32)
            n150 = Subtract(x=w128, y=w134) -> (x-y=w135:u32)
            n151 = case shown="2" w137 {
              selector: w137 -> [_ w149]
              tunnel: w136 -> [_ w150]
              tunnel: w135 -> [_ w147]
              frame 0, Default {
              }
              frame 2 {
                n152 = global read "Globals.vi" "PIXEL"() -> (w145:u32)
                n153 = To Long Integer(number=w145) -> (32bit integer=w146:i32)
                n154 = Initialize Array(u16 100, w146) -> (w152:u16[])
                n155 = call "ReturnFrame.vi"("Data Values In"=w152, "curr_nob"=w147, "curr_nos"=w150, "Drv"=w149) -> ("Data Values Out"=→"Signalverlaufgraph 2":u16[])  [unwired: 1 in]
              }
            }
            n156 = call "ReturnFrame.vi"("Data Values In"=w140, "curr_nob"=w135, "curr_nos"=w136, "Drv"=u32 1) -> ("Data Values Out"=→"Signalverlaufgraph":u16[])  [unwired: 1 in]
          }
          event "channel quick select (in hex)": Value Change {
            # "channel and camera select via quick select"
            n157 = event-data() -> ()  [unwired: 1 in, 6 out]
            n158 = flat-sequence {
              frame #0 {
                n159 = Number To Boolean Array(number="channel quick select (in hex)") -> (Boolean array=w200:bool[])
                n160 = Number To Boolean Array(number="channel quick select (in hex)") -> (Boolean array=w202:bool[])
                n161 = Number To Boolean Array(number="channel quick select (in hex)") -> (Boolean array=w192:bool[])
                n162 = Number To Boolean Array(number="channel quick select (in hex)") -> (Boolean array=w198:bool[])
                n163 = Number To Boolean Array(number="channel quick select (in hex)") -> (Boolean array=w194:bool[])
                n164 = Number To Boolean Array(number="channel quick select (in hex)") -> (Boolean array=w196:bool[])
                n165 = Number To Boolean Array(number="channel quick select (in hex)") -> (Boolean array=w188:bool[])
                n166 = Number To Boolean Array(number="channel quick select (in hex)") -> (Boolean array=w190:bool[])
                n167 = Index Array(array=w200, index=6) -> (element=w174:bool)
                n168 = Index Array(array=w202, index=7) -> (element=w173:bool)
                n169 = Index Array(array=w192, index=1) -> (element=w186:bool)
                n170 = Index Array(array=w198, index=5) -> (element=w178:bool)
                n171 = Index Array(array=w194, index=3) -> (element=w183:bool)
                n172 = Index Array(array=w196, index=4) -> (element=w179:bool)
                n173 = Index Array(array=w188, index=0) -> (element=w187:bool)
                n174 = Index Array(array=w190, index=2) -> (element=w184:bool)
                n175 = Or(x=w174, y=w173) -> (x .or. y?=w175:bool)
                n176 = Or(x=w179, y=w178) -> (x .or. y?=w177:bool)
                n177 = Or(x=w187, y=w186) -> (x .or. y?=w185:bool)
                n178 = Or(x=w184, y=w183) -> (x .or. y?=w182:bool)
                n179 = Build Array(w185) -> (w181:bool[])
                n180 = Build Array (concatenate)(w181, w182) -> (w180:bool[])
                n181 = Build Array (concatenate)(w180, w177) -> (w176:bool[])
                n182 = Build Array (concatenate)(w176, w175) -> (w172:bool[])
                n183 = property on="CHA 4" class="Bool (strict)"("Value"=w174) -> ()  [unwired: 2 in, 2 out]
                n184 = property on="CHB 4" class="Bool (strict)"("Value"=w173) -> ()  [unwired: 2 in, 2 out]
                n185 = property on="CHB 1" class="Bool (strict)"("Value"=w186) -> ()  [unwired: 2 in, 2 out]
                n186 = property on="CHB 3" class="Bool (strict)"("Value"=w178) -> ()  [unwired: 2 in, 2 out]
                n187 = property on="CHB 2" class="Bool (strict)"("Value"=w183) -> ()  [unwired: 2 in, 2 out]
                n188 = property on="CHA 3" class="Bool (strict)"("Value"=w179) -> ()  [unwired: 2 in, 2 out]
                n189 = property on="CHA 1" class="Bool (strict)"("Value"=w187) -> ()  [unwired: 2 in, 2 out]
                n190 = property on="CHA 2" class="Bool (strict)"("Value"=w184) -> ()  [unwired: 2 in, 2 out]
                n191 = Number To Boolean Array(number="channel quick select (in hex)") -> (Boolean array=w216:bool[])
                n192 = Number To Boolean Array(number="channel quick select (in hex)") -> (Boolean array=w218:bool[])
                n193 = Number To Boolean Array(number="channel quick select (in hex)") -> (Boolean array=w208:bool[])
                n194 = Number To Boolean Array(number="channel quick select (in hex)") -> (Boolean array=w214:bool[])
                n195 = Number To Boolean Array(number="channel quick select (in hex)") -> (Boolean array=w210:bool[])
                n196 = Number To Boolean Array(number="channel quick select (in hex)") -> (Boolean array=w212:bool[])
                n197 = Number To Boolean Array(number="channel quick select (in hex)") -> (Boolean array=w204:bool[])
                n198 = Number To Boolean Array(number="channel quick select (in hex)") -> (Boolean array=w206:bool[])
                n199 = Index Array(array=w216, index=14) -> (element=w158:bool)
                n200 = Index Array(array=w218, index=15) -> (element=w157:bool)
                n201 = Index Array(array=w208, index=9) -> (element=w169:bool)
                n202 = Index Array(array=w214, index=13) -> (element=w159:bool)
                n203 = Index Array(array=w210, index=11) -> (element=w167:bool)
                n204 = Index Array(array=w212, index=12) -> (element=w160:bool)
                n205 = Index Array(array=w204, index=8) -> (element=w170:bool)
                n206 = Index Array(array=w206, index=10) -> (element=w168:bool)
                n207 = Or(x=w170, y=w169) -> (x .or. y?=w171:bool)
                n208 = Or(x=w160, y=w159) -> (x .or. y?=w163:bool)
                n209 = Or(x=w168, y=w167) -> (x .or. y?=w165:bool)
                n210 = Or(x=w158, y=w157) -> (x .or. y?=w161:bool)
                n211 = Build Array (concatenate)(w172, w171) -> (w166:bool[])
                n212 = Build Array (concatenate)(w166, w165) -> (w164:bool[])
                n213 = Build Array (concatenate)(w164, w163) -> (w162:bool[])
                n214 = Build Array (concatenate)(w162, w161) -> (w153:bool[])
                n215 = property on="CHA 8" class="Bool (strict)"("Value"=w158) -> ()  [unwired: 2 in, 2 out]
                n216 = property on="CHB 8" class="Bool (strict)"("Value"=w157) -> ()  [unwired: 2 in, 2 out]
                n217 = property on="CHB 5" class="Bool (strict)"("Value"=w169) -> ()  [unwired: 2 in, 2 out]
                n218 = property on="CHB 7" class="Bool (strict)"("Value"=w159) -> ()  [unwired: 2 in, 2 out]
                n219 = property on="CHB 6" class="Bool (strict)"("Value"=w167) -> ()  [unwired: 2 in, 2 out]
                n220 = property on="CHA 7" class="Bool (strict)"("Value"=w160) -> ()  [unwired: 2 in, 2 out]
                n221 = property on="CHA 5" class="Bool (strict)"("Value"=w170) -> ()  [unwired: 2 in, 2 out]
                n222 = property on="CHA 6" class="Bool (strict)"("Value"=w168) -> ()  [unwired: 2 in, 2 out]
                n223 = Number To Boolean Array(number="channel quick select (in hex)") -> (Boolean array=w226:bool[])
                n224 = global read "Globals.vi" "maddr of CC"() -> (w220:u8)
                n225 = Boolean To (0,1)(Boolean=w226) -> (0, 1=w222:i16[])
                n226 = global read "Globals.vi" "reg_addr-CH_select"() -> (w221:u8)
                n227 = Boolean To (0,1)(Boolean=w153) -> (0, 1=w156:i16[])
                n228 = Add Array Elements(numeric array=w222) -> (sum=w224:i16)
                n229 = Add Array Elements(numeric array=w156) -> (sum=w155:i16)
                n230 = To Unsigned Byte Integer(number=w224) -> (unsigned 8bit integer=w223:u8)
                n231 = To Unsigned Byte Integer(number=w155) -> (unsigned 8bit integer=w154:u8)
                n232 = call "SendFLCam.vi"("madr"=w220, "data"="channel quick select (in hex)", "adadr"=w221) -> ()
                n233 = global write "Globals.vi" "devices_amount"(w154) -> ()
                n234 = global write "Globals.vi" "cams_amount"(w223) -> ()
              }
              frame #1 {
                # "refresh nos for triggering MB calc"
                n235 = global read "Globals.vi" "devices_amount"() -> (w228:u8)
                n236 = global read "Globals.vi" "cams_amount"() -> (w229:u8)
                n237 = property on="no.of blocks (nob)\npress enter" class="DigNum (strict)"() -> ("Value"=w227:u32)  [unwired: 2 in, 2 out]
                n238 = property on="amount of cams" class="DigNum (strict)"("Value"=w229) -> ()  [unwired: 2 in, 2 out]
                n239 = property on="no.of blocks (nob)\npress enter" class="DigNum (strict)"("Val(Sgnl)"=w227) -> ()  [unwired: 2 in, 2 out]
                n240 = property on="amount of devices" class="DigNum (strict)"("Value"=w228) -> ()  [unwired: 2 in, 2 out]
              }
            }
          }
          event "CHA 1", "CHB 1", "CHA 2", "CHB 2", "CHA 3", "CHB 3", "CHA 4", "CHB 4", "CHA 5", "CHB 5", "CHA 6", "CHB 6", "CHA 7", "CHB 7", "CHA 8", "CHB 8": Value Change {
            # "channel and camera select via switches"
            n241 = event-data() -> ()  [unwired: 1 in, 6 out]
            n242 = flat-sequence {
              frame #0 {
                n243 = Or(x="CHB 4", y="CHA 4") -> (x .or. y?=w242:bool)
                n244 = Or(x="CHB 3", y="CHA 3") -> (x .or. y?=w244:bool)
                n245 = Build Array("CHA 1") -> (w269:bool[])
                n246 = Build Array (concatenate)(w269, "CHB 1") -> (w270:bool[])
                n247 = Or(x="CHB 2", y="CHA 2") -> (x .or. y?=w246:bool)
                n248 = Build Array (concatenate)(w270, "CHA 2") -> (w271:bool[])
                n249 = Build Array (concatenate)(w271, "CHB 2") -> (w272:bool[])
                n250 = Build Array (concatenate)(w272, "CHA 3") -> (w273:bool[])
                n251 = Build Array (concatenate)(w273, "CHB 3") -> (w274:bool[])
                n252 = Build Array (concatenate)(w274, "CHA 4") -> (w275:bool[])
                n253 = Build Array (concatenate)(w275, "CHB 4") -> (w276:bool[])
                n254 = Or(x="CHA 1", y="CHB 1") -> (x .or. y?=w248:bool)
                n255 = Build Array(w248) -> (w247:bool[])
                n256 = Build Array (concatenate)(w247, w246) -> (w245:bool[])
                n257 = Build Array (concatenate)(w245, w244) -> (w243:bool[])
                n258 = Build Array (concatenate)(w243, w242) -> (w241:bool[])
                n259 = Build Array (concatenate)(w276, "CHA 5") -> (w277:bool[])
                n260 = Build Array (concatenate)(w277, "CHB 5") -> (w278:bool[])
                n261 = Build Array (concatenate)(w278, "CHA 6") -> (w279:bool[])
                n262 = Build Array (concatenate)(w279, "CHB 6") -> (w280:bool[])
                n263 = Build Array (concatenate)(w280, "CHA 7") -> (w281:bool[])
                n264 = Build Array (concatenate)(w281, "CHB 7") -> (w282:bool[])
                n265 = Build Array (concatenate)(w282, "CHA 8") -> (w283:bool[])
                n266 = Build Array (concatenate)(w283, "CHB 8") -> (w268:bool[])
                n267 = Or(x="CHA 5", y="CHB 5") -> (x .or. y?=w240:bool)
                n268 = Or(x="CHB 6", y="CHA 6") -> (x .or. y?=w238:bool)
                n269 = Or(x="CHA 7", y="CHB 7") -> (x .or. y?=w236:bool)
                n270 = Or(x="CHA 8", y="CHB 8") -> (x .or. y?=w234:bool)
                n271 = Boolean To (0,1)(Boolean=w268) -> (0, 1=w267:i16[])
                n272 = Boolean Array To Number(Boolean array=w268) -> (number=w284:u32)
                n273 = Build Array (concatenate)(w241, w240) -> (w239:bool[])
                n274 = Build Array (concatenate)(w239, w238) -> (w237:bool[])
                n275 = Build Array (concatenate)(w237, w236) -> (w235:bool[])
                n276 = Build Array (concatenate)(w235, w234) -> (w233:bool[])
                n277 = Add Array Elements(numeric array=w267) -> (sum=w265:i16)
                n278 = To Unsigned Word Integer(number=w284) -> (unsigned 16bit integer=w285:u16)
                n279 = To Unsigned Byte Integer(number=w265) -> (unsigned 8bit integer=w266:u8)
                n280 = Boolean To (0,1)(Boolean=w233) -> (0, 1=w232:i16[])
                n281 = Add Array Elements(numeric array=w232) -> (sum=w231:i16)
                n282 = global write "Globals.vi" "cams_amount"(w266) -> ()
                n283 = property on="channel quick select (in hex)" class="DigNum (strict)"("Value"=w285) -> ()  [unwired: 2 in, 2 out]
                n284 = To Unsigned Byte Integer(number=w231) -> (unsigned 8bit integer=w230:u8)
                n285 = global write "Globals.vi" "devices_amount"(w230) -> ()
              }
              frame #1 {
                # "refresh nos for triggering MB calc"
                n286 = global read "Globals.vi" "devices_amount"() -> (→"amount of devices":u8)
                n287 = global read "Globals.vi" "cams_amount"() -> (→"amount of cams":u8)
                n288 = global read "Globals.vi" "maddr of CC"() -> (w289:u8)
                n289 = global read "Globals.vi" "reg_addr-CH_select"() -> (w290:u8)
                n290 = property on="channel quick select (in hex)" class="DigNum (strict)"() -> ("Value"=w291:u16)  [unwired: 2 in, 2 out]
                n291 = call "SendFLCam.vi"("madr"=w289, "data"=w291, "adadr"=w290) -> ()
                n292 = property on="no.of samples (nos)" class="DigNum (strict)"() -> ("Value"=w286:u32)  [unwired: 2 in, 2 out]
                n293 = property on="no.of samples (nos)" class="DigNum (strict)"("Val(Sgnl)"=w286) -> ()  [unwired: 2 in, 2 out]
              }
            }
          }
          event "no.of samples (nos)", "no.of blocks (nob)\npress enter", "exposuretime[ms]": Value Change {
            # "calculation of MB RAM an SEC and setting scale max"
            # "MB"
            # "ushort"
            n294 = event-data() -> ()  [unwired: 1 in, 7 out]
            n295 = global read "Globals.vi" "PIXEL"() -> (w317:u32)
            n296 = Multiply(x="no.of samples (nos)", y=w317) -> (x*y=w315:u32)
            n297 = Multiply(x=w315, y=u32 2) -> (x*y=w295:u32)
            n298 = global read "Globals.vi" "boards"() -> (w316:u32)
            n299 = global read "Globals.vi" "cams_amount"() -> (w294:u8)
            n300 = global read "Globals.vi" "nos"() -> (w299:u32)
            n301 = global read "Globals.vi" "nob"() -> (w297:u32)
            n302 = To Unsigned Long Integer(number=w294) -> (unsigned 32bit integer=w293:u32)
            n303 = Multiply(x=w293, y=w295) -> (x*y=w292:u32)
            n304 = Multiply(x=w292, y=w316) -> (x*y=w305:u32)
            n305 = To Double Precision Float(number=w305) -> (double precision float=w304:dbl)
            n306 = To Double Precision Float(number=w299) -> (double precision float=w298:dbl)
            n307 = Divide(x=w304, y=1048576.0) -> (x/y=w307:dbl)
            n308 = To Double Precision Float(number=w297) -> (double precision float=w296:dbl)
            n309 = To Double Precision Float(number="no.of blocks (nob)\npress enter") -> (double precision float=w302:dbl)
            n310 = property on="sample" class="Slide (strict)"("Scale.Maximum"=w298) -> ()  [unwired: 2 in, 2 out]
            n311 = property on="block" class="Slide (strict)"("Scale.Maximum"=w296) -> ()  [unwired: 2 in, 2 out]
            n312 = Multiply(x=w307, y=w302) -> (x*y=→"MB RAM":dbl)
            n313 = global write "Globals.vi" "nos"("no.of samples (nos)") -> ()
            n314 = Multiply(x="no.of samples (nos)", y="no.of blocks (nob)\npress enter") -> (x*y=w300:u32)
            n315 = global write "Globals.vi" "nob"("no.of blocks (nob)\npress enter") -> ()
            n316 = To Double Precision Float(number=w300) -> (double precision float=w301:dbl)
            n317 = global write "Globals.vi" "exp time"("exposuretime[ms]") -> ()
            n318 = Multiply(x="exposuretime[ms]", y=w301) -> (x*y=w313:dbl)
            n319 = Divide(x=w313, y=1000.0) -> (x/y=→"SEC":dbl)
          }
          event "stop all": Value Change {
            # "exit"
            n320 = event-data() -> ()  [unwired: 1 in, 6 out]
            n321 = stacked-sequence {
              tunnel: [_ TRUE] -> w318
              frame #0 {
                n322 = call "FFStop.vi"() -> ()  [unwired: 1 in]
              }
              frame #1 {
                # "do not omit, or next call of driver will go wrong."
                n323 = call "Exit.vi"() -> ()  [unwired: 1 in]
              }
            }
          }
          event "rms_pixel": Value Change {
            # "one array with all values (except first 10)\nat index Pixel from all blocks"
            n324 = event-data() -> ()  [unwired: 1 in, 6 out]
            n325 = global read "Globals.vi" "nos"() -> (w324:u32)
            n326 = global read "Globals.vi" "nob"() -> (w325:u32)
            n327 = for {
              N: w325 -> [_]
              tunnel: w324 -> [w326]
              tunnel: [w328] -> w321 mode=concatenating
              i -> [w332]
              # "delete first 10 values"
              # "array of all values\nat index Pixel"
              n328 = To Long Integer(number=w326) -> (32bit integer=w327:i32)
              n329 = for {
                N: w327 -> [_]
                tunnel: w332 -> [w337]
                tunnel: [w341] -> w329 mode=indexing
                i -> [w339]
                # "use only value at index \"Pixel\""
                # "init array of size PIXEL\nwith value 100"
                n330 = global read "Globals.vi" "PIXEL"() -> (w333:u32)
                n331 = To Long Integer(number=w333) -> (32bit integer=w334:i32)
                n332 = To Unsigned Long Integer(number=w337) -> (unsigned 32bit integer=w338:u32)
                n333 = To Unsigned Long Integer(number=w339) -> (unsigned 32bit integer=w340:u32)
                n334 = Initialize Array(u16 100, w334) -> (w343:u16[])
                n335 = call "ReturnFrame.vi"("Data Values In"=w343, "curr_nob"=w338, "curr_nos"=w340, "Drv"=u32 1) -> ("Data Values Out"=w342:u16[])  [unwired: 1 in]
                n336 = To Long Integer(number="rms_pixel") -> (32bit integer=w335:i32)
                n337 = Index Array(array=w342, index=w335) -> (element=w341:u16)
              }
              n338 = Delete From Array(array=w329, length=10, index=0) -> (array with subset deleted=w328:u16[])  [unwired: 1 out]
            }
            n339 = To Double Precision Float(number=w321) -> (double precision float=w320:dbl[])
            n340 = call <vilib>:"Std Deviation and Variance.vi"("X"=w320) -> ("mean"=→"mean":dbl, "standard deviation"=→"tRMS":dbl)  [unwired: 1 in, 1 out]
          }
        }
      }
    }
  }
  n341 = property on="sample" class="Slide (strict)"("DisabledEnum"=w1) -> ()  [unwired: 2 in, 2 out]
  n342 = property on="start" class="Bool (strict)"("DisabledEnum"=w1) -> ()  [unwired: 2 in, 2 out]
  n343 = property on="block" class="Slide (strict)"("DisabledEnum"=w1) -> ()  [unwired: 2 in, 2 out]
